vi "Read Boolean.vi"(8 "error in (no error)":errorcluster, 9 "section":string, 10 "keys":string[](array[string]), 11 "FileConfig in":refnum<class "FileConfig.lvclass">) -> (0 "error out":errorcluster, 1 "Found?":bool, 2 "Found Booleans":bool[](array[boolean]), 3 "FileConfig out":refnum<class "FileConfig.lvclass">)   [LabVIEW 2018, in "Config.lvlib" / "FileConfig.lvclass"]
doc: "Use this VI to read IDs from the File"
uses:
  FileConfig.lvclass
  Config/Controls/KeyType.ctl
  Config.lvclass
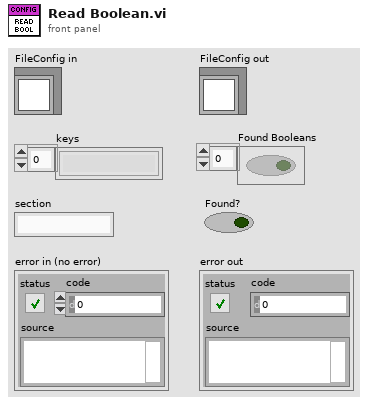
[diagram p1: front panel]
types:
  T1 = typedef "Config.lvlib/Config.lvclass/KeyType.ctl" = enum16{"dbl", "path", "string ", "u32", "i32", "boolean"}
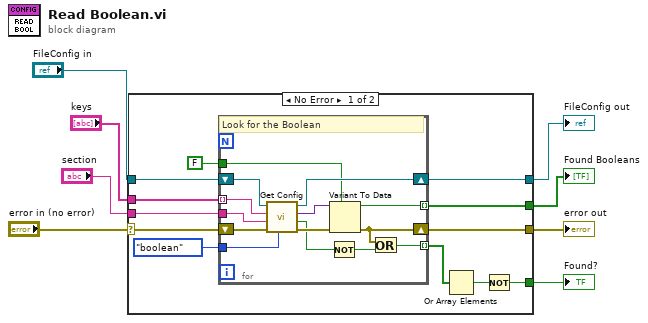
[diagram p0: block diagram]
diagram:
  n1 = case shown="No Error" "error in (no error)" {
    selector: "error in (no error)" -> [w20 w36]
    tunnel: "FileConfig in" -> [w19 w35]
    tunnel: [w18 w36] -> w6
    tunnel: [w17 w35] -> w5
    tunnel: [w16 _] -> w4
    tunnel: [w13 _] -> w3
    tunnel: "keys" -> [w10 _]
    tunnel: "section" -> [w9 _]
    frame No Error {
      n2 = for {
        shift-right: [w33] -> w17
        shift-left: w19 -> [w34]
        shift-right: [w24] -> w18
        shift-left: w20 -> [w32]
        tunnel: w9 -> [w30]
        tunnel: w10 -> [w29] mode=indexing
        tunnel: KeyType."boolean" -> [w28]
        tunnel: FALSE -> [w26]
        tunnel: [w25] -> w13 mode=indexing
        tunnel: [w21] -> w14 mode=indexing
        # "Look for the Boolean"
        n3 = call-dynamic "Get Config.vi"(6:w28, "error in (no error)"=w32, "section"=w30, "key"=w29, "FileConfig in"=w34) -> ("error out"=w31:errorcluster, "found?"=w23:bool, "Data"=w27:variant, "FileConfig out"=w33:refnum<class "FileConfig.lvclass">)  [unwired: 3 in]
        n4 = Not(x=w23) -> (.not. x?=w22:bool)
        n5 = Variant To Data(error in=w31, type=w26, Variant=w27) -> (data=w25:bool, error out=w24:errorcluster)
        n6 = Or(x=w24, y=w22) -> (x .or. y?=w21:bool)
      }
      n7 = Or Array Elements(Boolean array=w14) -> (logical OR=w15:bool)
      n8 = Not(x=w15) -> (.not. x?=w16:bool)
    }
    frame Error {
    }
  }
  "error out" <- w6
  "FileConfig out" <- w5
  "Found?" <- w4
  "Found Booleans" <- w3
